vi "Update_Message.vi"(8 "error in (no error)":errorcluster, 10 "Message":T1, 11 "ATM_UI_Controller in":refnum<class "ATM_UI_Controller.lvclass">) -> (0 "error out":errorcluster, 3 "ATM_UI_Controller out":refnum<class "ATM_UI_Controller.lvclass">)   [LabVIEW 2025, in "ATM_UI_Controller.lvlib" / "ATM_UI_Controller.lvclass"]
uses:
  ATM_UI_Controller.lvclass
  ATM_UI_Controller.lvclass/ATM_UI_Controller.ctl
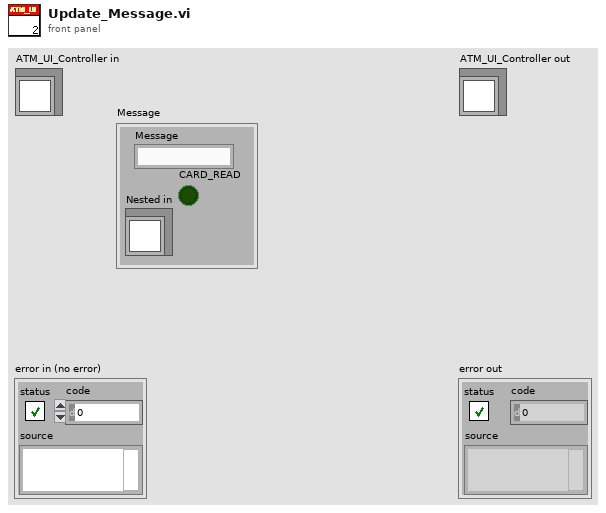
[diagram p1: front panel]
types:
  T1 = cluster{"Message":string, "CARD_READ":bool, "Nested in":refnum<class "ATM_UI_Controller.lvclass">}
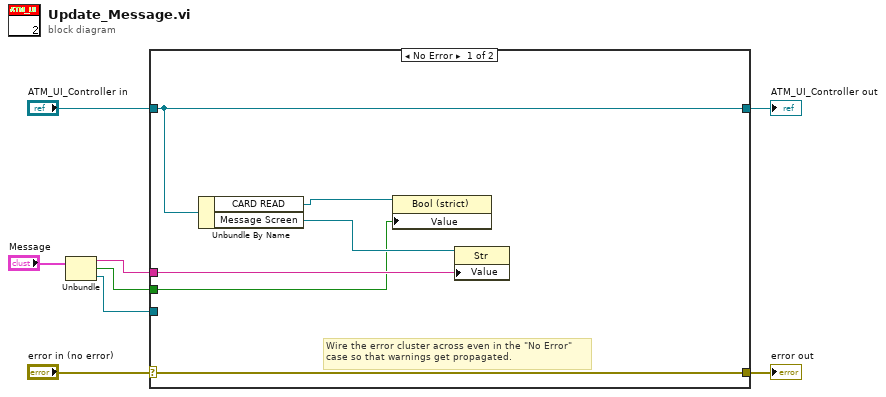
[diagram p0: block diagram]
diagram:
  n1 = Unbundle("Message") -> ("Message"=w3:string, "CARD_READ"=w2:bool, "Nested in"=w1:refnum<class "ATM_UI_Controller.lvclass">)
  n2 = case shown="No Error" "error in (no error)" {
    selector: "error in (no error)" -> [w14 w16]
    tunnel: [w14 w16] -> w7
    tunnel: [w9 w15] -> w5
    tunnel: "ATM_UI_Controller in" -> [w9 w15]
    tunnel: w3 -> [w12 _]
    tunnel: w2 -> [w10 _]
    tunnel: w1 -> [_ _]
    frame No Error {
      # "Wire the error cluster across even in the \"No Error\"\ncase so that warnings get propagated."
      n3 = Unbundle By Name(w9) -> ("CARD READ"=w11:refnum<vi>, "Message Screen"=w13:refnum<vi>)
      n4 = property class="Bool (strict)"(reference=w11, "Value"=w10) -> ()  [unwired: 1 in, 2 out]
      n5 = property class="Str"(reference=w13, "Value"=w12) -> ()  [unwired: 1 in, 2 out]
    }
    frame Error {
    }
  }
  "error out" <- w7
  "ATM_UI_Controller out" <- w5
